vi "Init Module.vi"(8 "error in (no error)":errorcluster, 11 "Singleton Module Admin in":refnum<class "Delacor_lib_QMH_Module Admin.lvclass">) -> (0 "error out":errorcluster, 2 "Configuracion Request Events":T1, 3 "Singleton Module Admin out":refnum<class "Delacor_lib_QMH_Module Admin.lvclass">)   [LabVIEW 2019, in "Configuracion.lvlib"]
doc: "Initialize the module by creating Broadcast Events, Request Events, and synchronization rendezvous.\n_____\nBased on Delacor QMH Project Template 5.0.0.82."
uses:
  Configuracion.lvlib
  <vilib>/Delacor/Delacor QMH/Libraries/Module Admin_class/Delacor_lib_QMH_Module Admin.lvclass
  Request Events--cluster.ctl
  Stop Argument--cluster.ctl
  Show Panel Argument--cluster.ctl
  Hide Panel Argument--cluster.ctl
  Get Module Execution Status Argument--cluster.ctl
  Show Diagram Argument--cluster.ctl
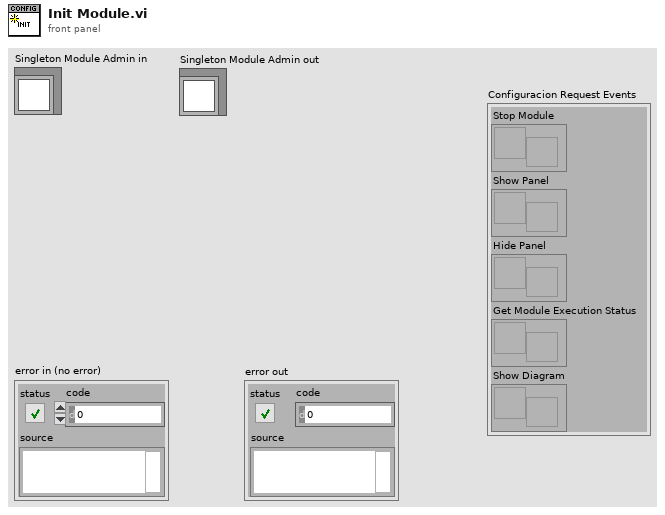
[diagram p1: front panel]
types:
  T1 = typedef "Configuracion.lvlib/Request Events--cluster.ctl" = cluster{"Stop Module":refnum<user-event>, "Show Panel":refnum<user-event>, "Hide Panel":refnum<user-event>, "Get Module Execution Status":refnum<user-event>, "Show Diagram":refnum<user-event>}
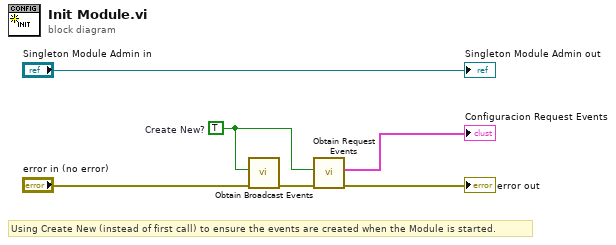
[diagram p0: block diagram]
diagram:
  w3 = TRUE  # Create New?
  # "Using Create New (instead of first call) to ensure the events are created when the Module is started."
  n1 = call "Obtain Broadcast Events.vi"("error in (no error)"="error in (no error)", "Create New? (F)"=w3) -> ("error out"=w6:errorcluster)  [unwired: 8 in, 1 out]
  n2 = call "Obtain Request Events.vi"("error in (no error)"=w6, "Create New? (F)"=w3) -> ("error out"=→"error out":errorcluster, "Configuracion Request Events"=→"Configuracion Request Events":T1)  [unwired: 8 in]
  "Singleton Module Admin out" <- "Singleton Module Admin in"
